vi "alpha_0.4.vi"() -> ()   [LabVIEW 2019]
panel:
  out "Congestionamento 2":bool
  in  "Rácio de entrada 2":dbl
  in  "Slide 2":dbl(slide) scale=0.0..10.0
  in  "Velocidade 2":dbl
  out "Vel3":bool
  out "Vel2":bool
  out "Vel1":bool
  out "RP1 3":bool
  out "GP1 3":bool
  out "G1 3":bool
  out "Y1 3":bool
  out "R1 3":bool
  out "RP1 2":bool
  out "GP1 2":bool
  out "G1 2":bool
  out "Y1 2":bool
  out "R1 2":bool
  out "RP1":bool
  out "GP1":bool
  out "G1":bool
  out "Y1":bool
  out "R1":bool
  in  "Rácio de entrada":dbl
  in  "Rácio de entrada 3":dbl
  out "Tempo no Vermelho":dbl caption="Elapsed Time (s)"
  out "Tempo no Verde + Amarelo":dbl caption="Elapsed Time (s)"
  out "Congestionamento 3":bool
  out "Congestionamento 1":bool
  in  "Slide 3":dbl(slide) scale=0.0..10.0
  in  "Slide 1":dbl(slide) scale=0.0..10.0
  in  "Caso de emergência":bool
  out "GreenP 2":bool
  out "RedP 2":bool
  out "GreenP 1":bool
  out "RedP 1":bool
  in  "Estado 2":dbl
  out "Velocidade excedida 3":bool
  in  "Velocidade 3":dbl
  out "RED 4":bool
  out "YELLOW 4":bool
  out "GREEN 4":bool
  out "Velocidade excedida 2":bool
  in  "Velocidade":dbl
  out "RED 3":bool
  out "YELLOW 3":bool
  out "GREEN 3":bool
  in  "stop":bool
  in  "Timer (s)":dbl
  # "Inputs"
  # "Inputs"
  # "Inputs"
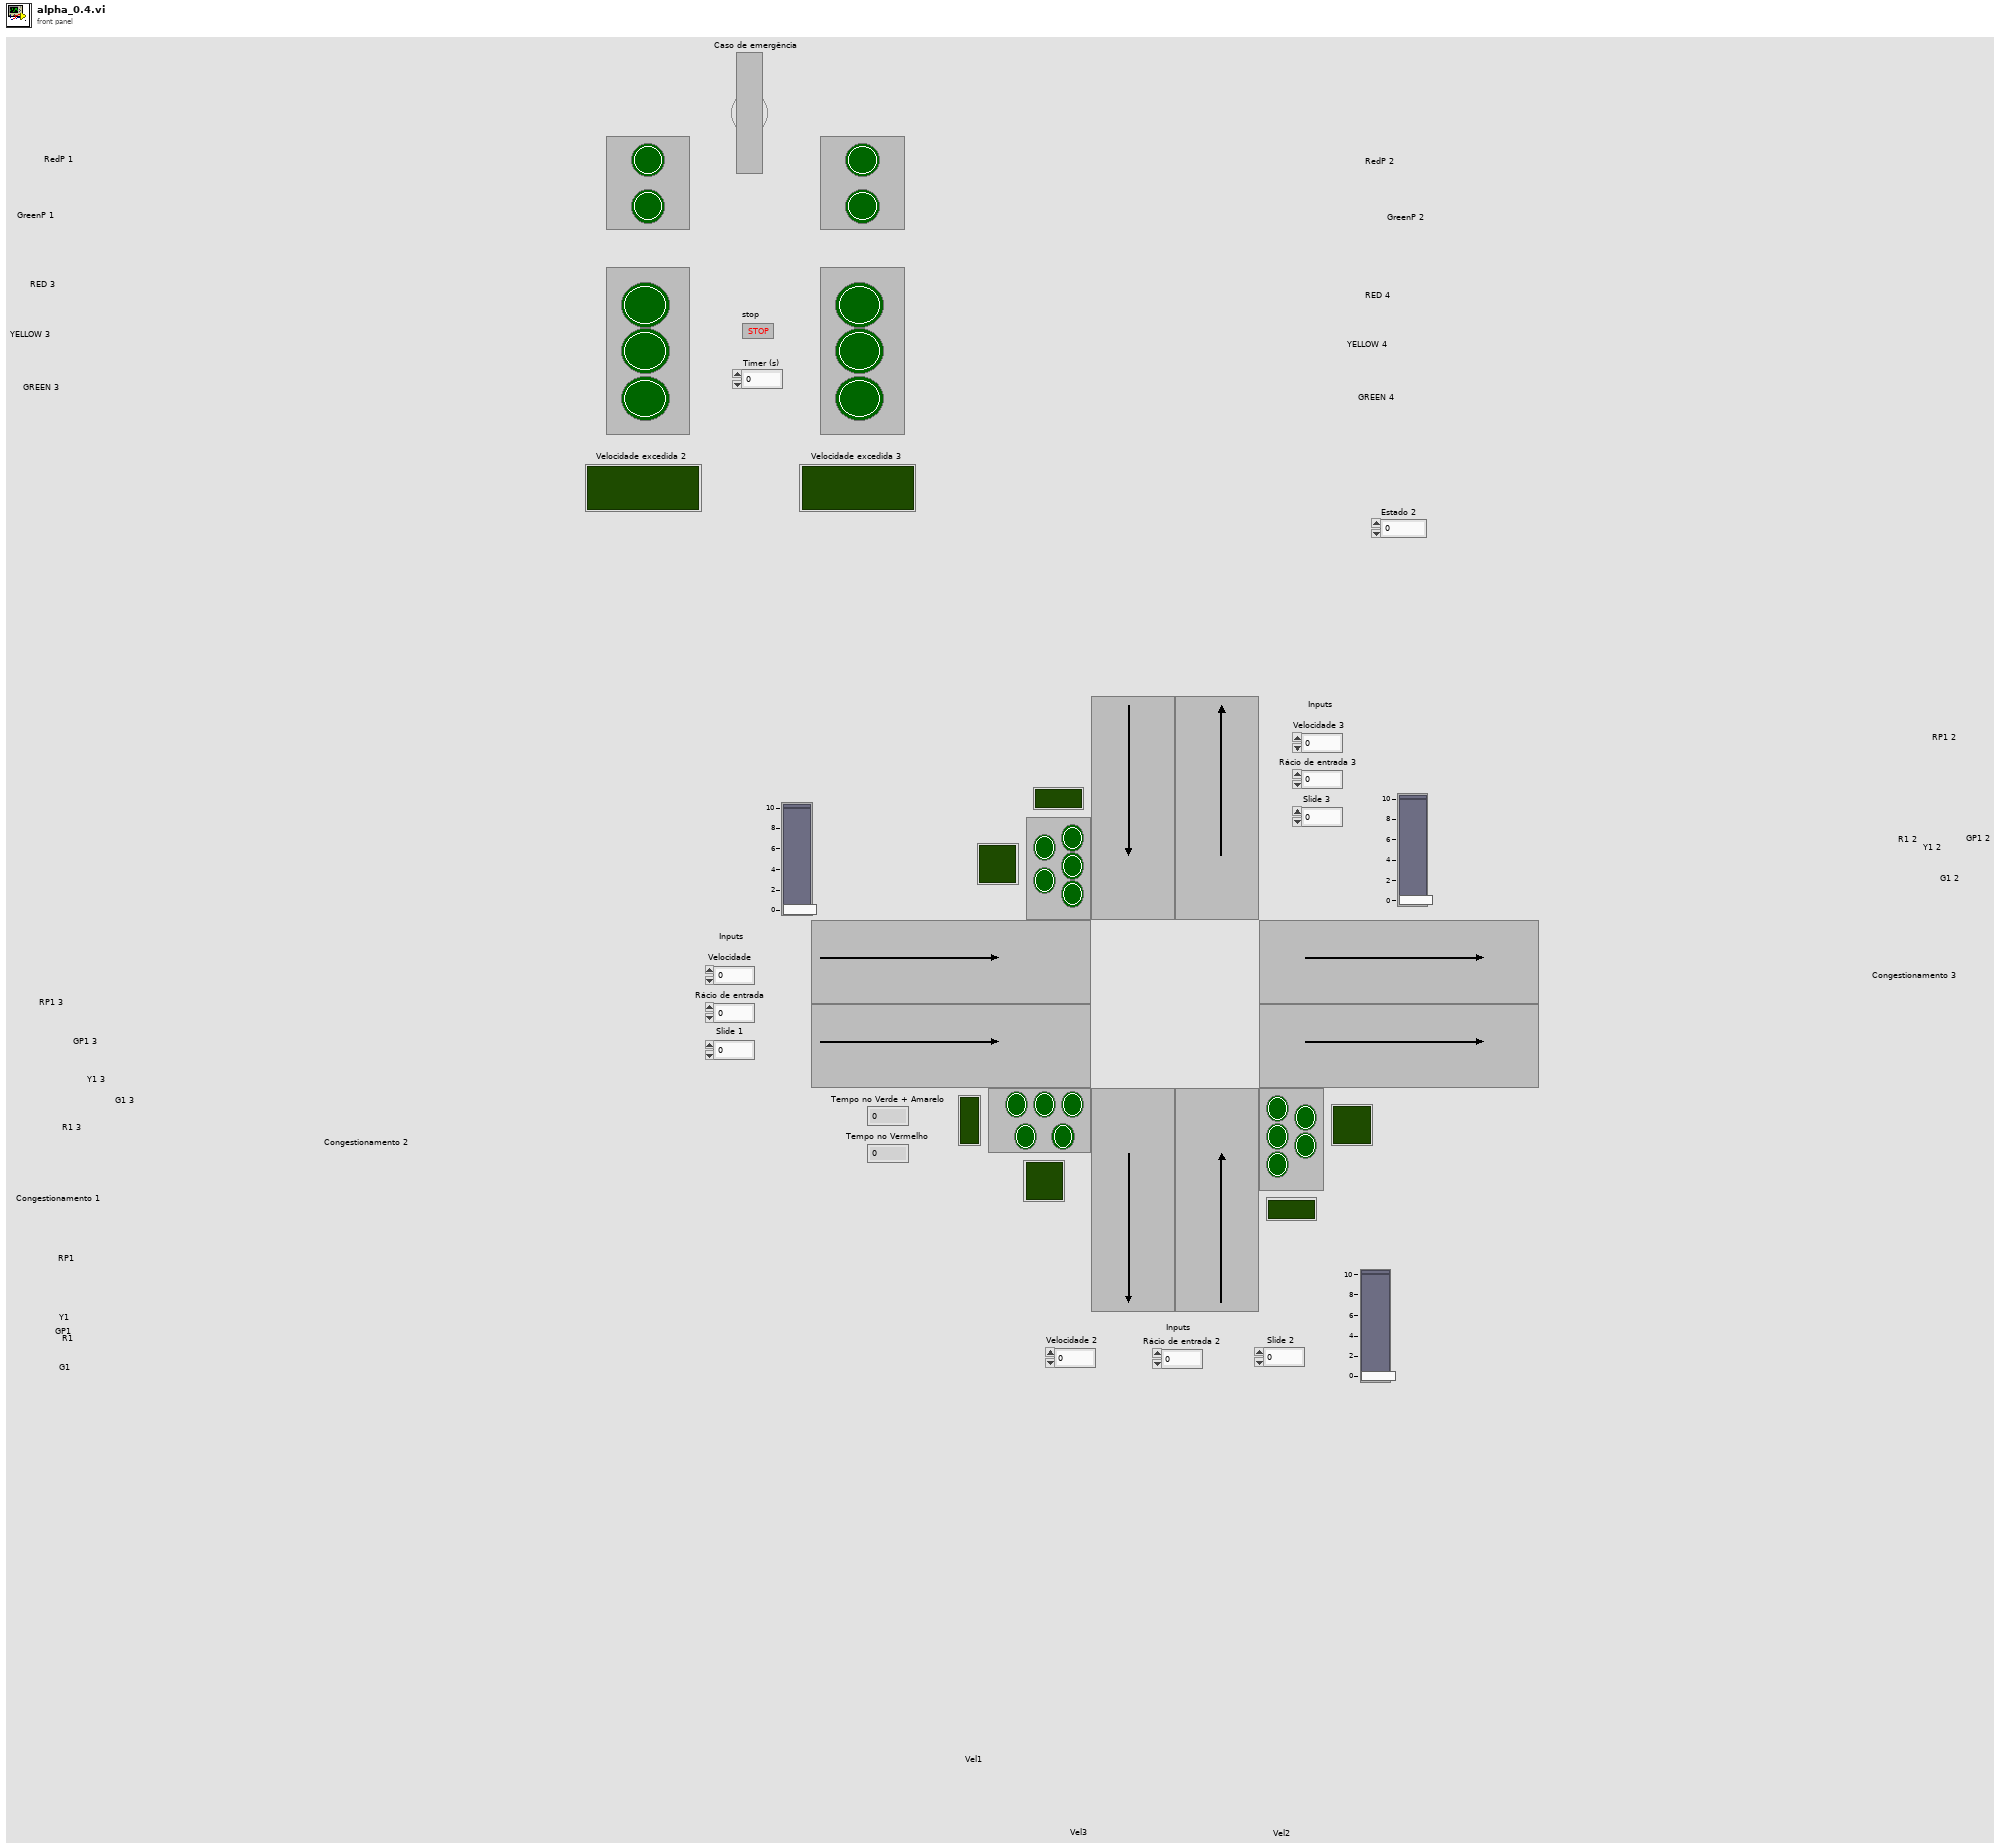
[diagram p1: front panel]
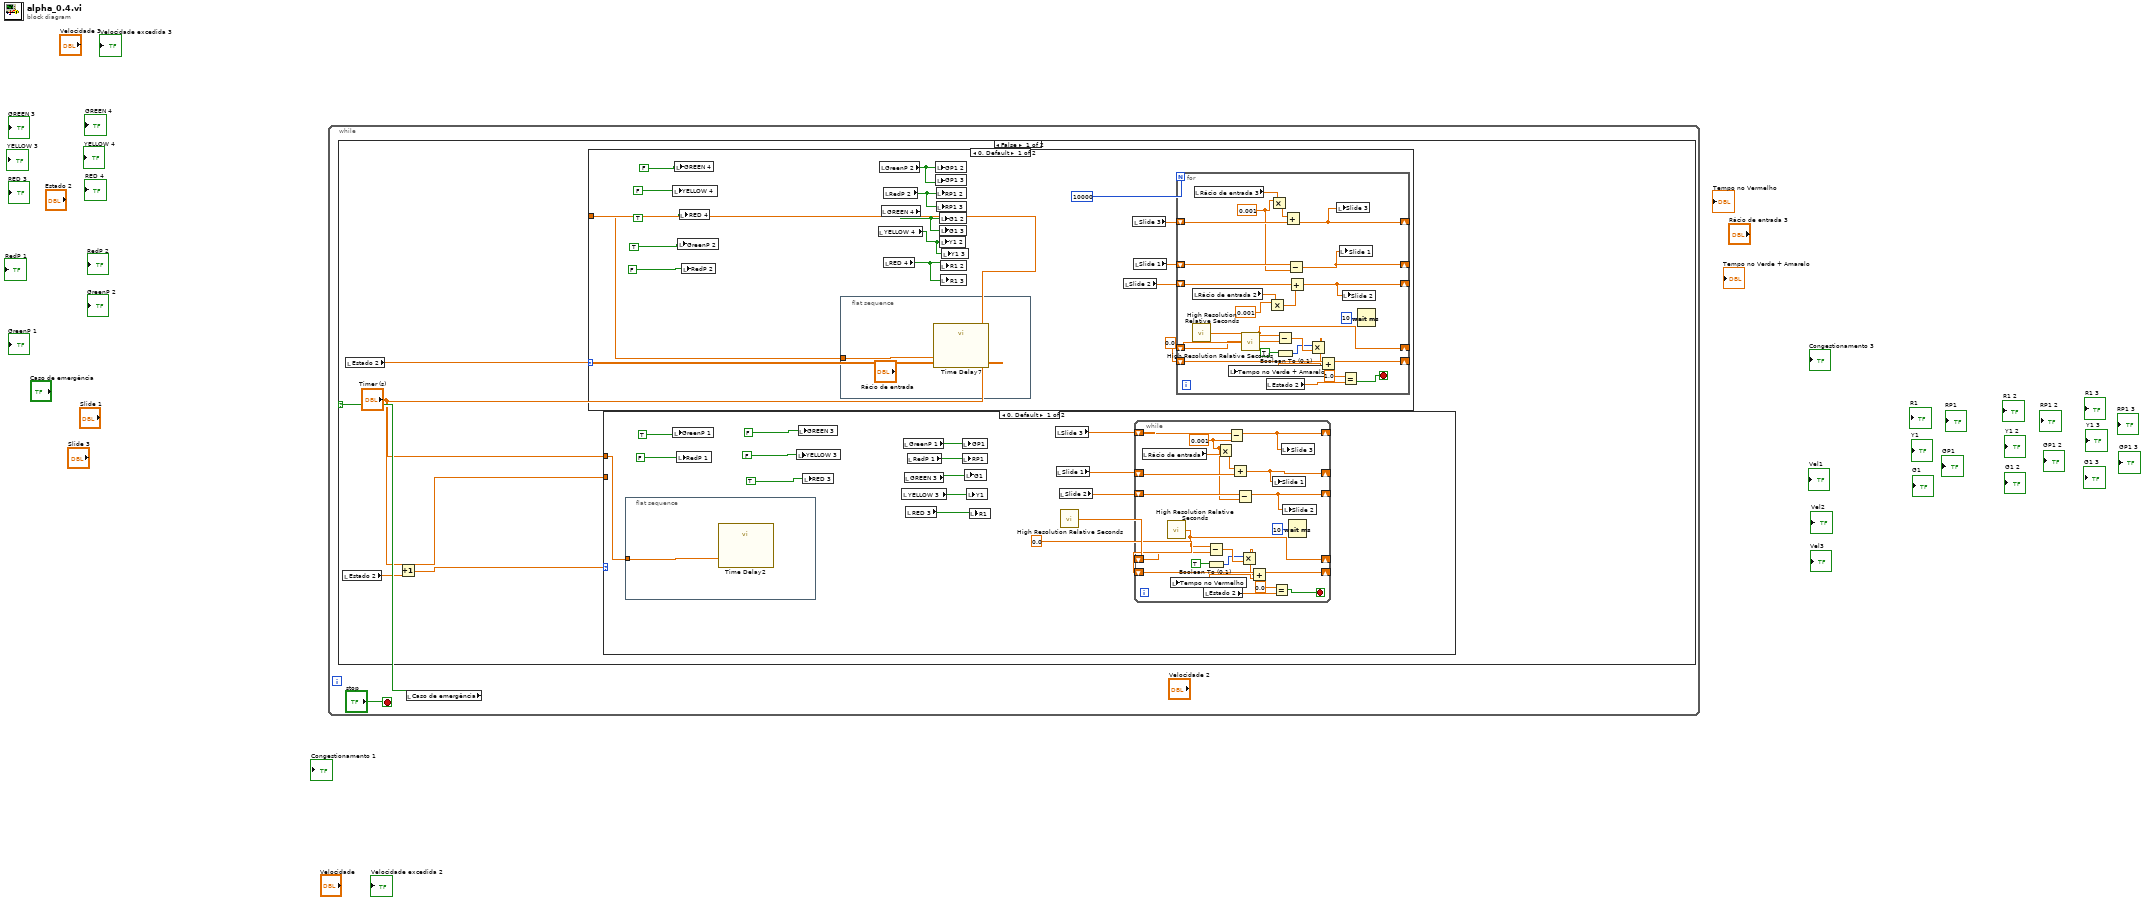
[diagram p0: block diagram]
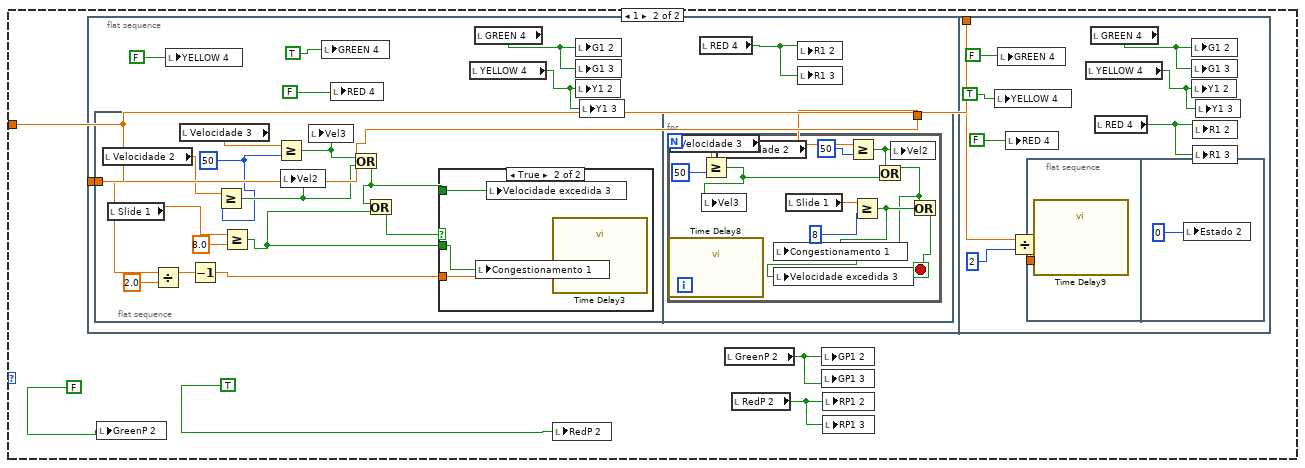
[diagram p2: hidden frame]
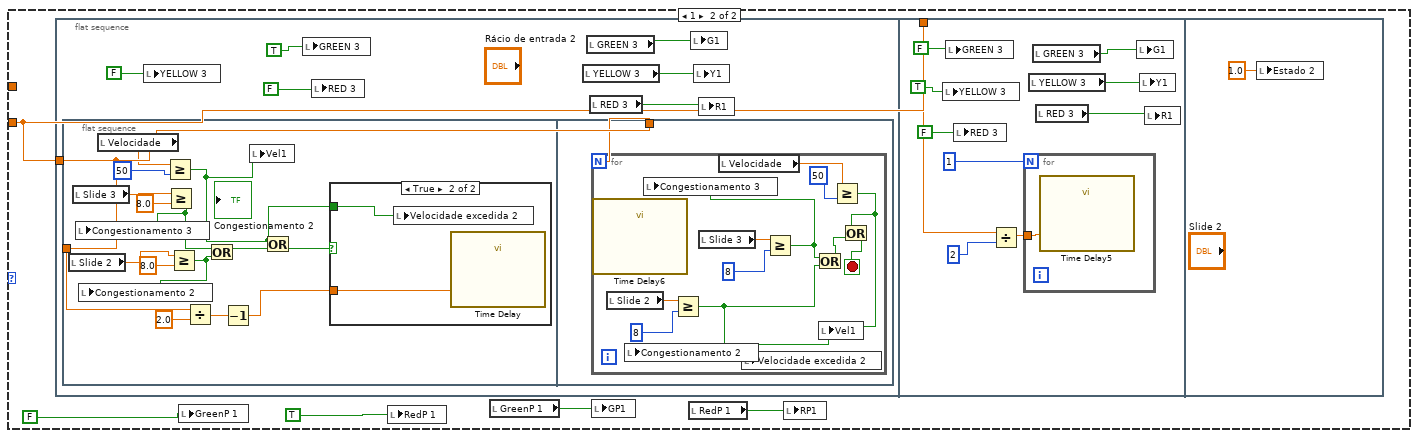
[diagram p4: hidden frame]
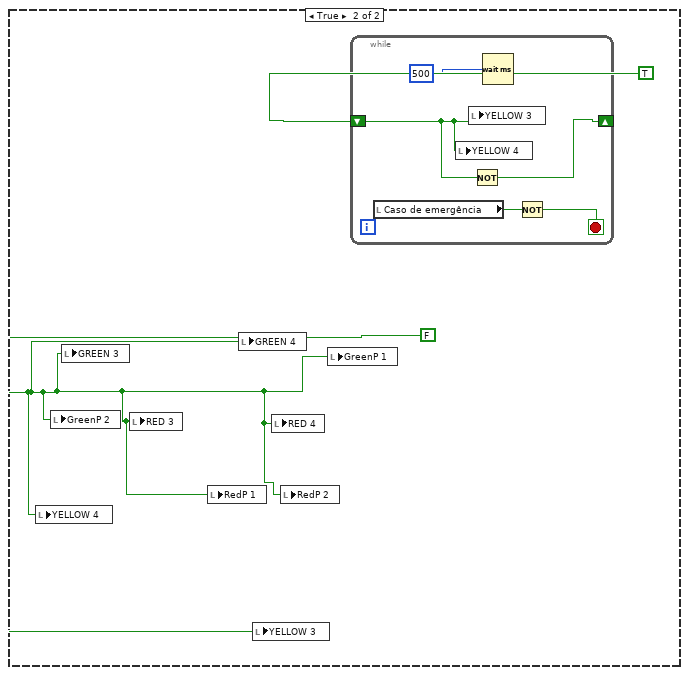
[diagram p6: hidden frame]
diagram:
  n1 = while {
    stop <- "stop" stop-if-true
    n2 = local read "Caso de emergência"() -> (w1:bool)
    n3 = case shown="False" w1 {
      frame False {
        n4 = local read "Estado 2"() -> (w6:dbl)
        n5 = local read "Estado 2"() -> (w4:dbl)
        n6 = Increment(x=w6) -> (x+1=w5:dbl)
        n7 = case shown="0, Default" w4 {
          tunnel: "Timer (s)" -> [w18 w53]
          frame 0, Default {
            n8 = local write "YELLOW 4"(FALSE) -> ()
            n9 = local write "GREEN 4"(FALSE) -> ()
            n10 = local write "GreenP 2"(TRUE) -> ()
            n11 = local write "RED 4"(TRUE) -> ()
            n12 = local write "RedP 2"(FALSE) -> ()
            n13 = flat-sequence {
              tunnel: w18 -> [w48]
              frame #0 {
                n14 = call "Time Delay7"("Delay Time (s)"=w48) -> ()  [unwired: 10 in, 1 out]
              }
            }
            n15 = local read "YELLOW 4"() -> (w9:bool)
            n16 = local read "GreenP 2"() -> (w12:bool)
            n17 = local read "GREEN 4"() -> (w10:bool)
            n18 = local read "RedP 2"() -> (w11:bool)
            n19 = local read "RED 4"() -> (w8:bool)
            n20 = local write "GP1 2"(w12) -> ()
            n21 = local write "GP1 3"(w12) -> ()
            n22 = local write "RP1 2"(w11) -> ()
            n23 = local write "RP1 3"(w11) -> ()
            n24 = local write "G1 2"(w10) -> ()
            n25 = local write "G1 3"(w10) -> ()
            n26 = local write "Y1 2"(w9) -> ()
            n27 = local write "R1 2"(w8) -> ()
            n28 = local write "R1 3"(w8) -> ()
            n29 = local write "Y1 3"(w9) -> ()
            n30 = local read "Slide 2"() -> (w7:dbl)
            n31 = local read "Slide 3"() -> (w13:dbl)
            n32 = local read "Slide 1"() -> (w14:dbl)
            n33 = call <vilib>:"High Resolution Relative Seconds.vi"() -> ("relative seconds"=w17:dbl)
            n34 = for {
              N: 10000 -> [_]
              shift-right: [w45] -> _
              shift-left: w17 -> [w46]
              shift-right: [w39] -> _
              shift-left: 0.0 -> [w44]
              shift-right: [w33] -> _
              shift-left: w13 -> [w35]
              shift-right: [w31] -> _
              shift-left: w14 -> [w30]
              shift-right: [w24] -> _
              shift-left: w7 -> [w28]
              stop <- w37 stop-if-true
              w29 = 0.001 ("x")
              n35 = local read "Rácio de entrada 2"() -> (w26:dbl)
              n36 = call <vilib>:"High Resolution Relative Seconds.vi"() -> ("relative seconds"=w45:dbl)
              n37 = local read "Rácio de entrada 3"() -> (w34:dbl)
              n38 = local read "Estado 2"() -> (w38:dbl)
              n39 = Multiply(x=0.001, y=w26) -> (x*y=w25:dbl)
              n40 = Multiply(x=w29, y=w34) -> (x*y=w32:dbl)
              n41 = Subtract(x=w45, y=w46) -> (x-y=w42:dbl)
              n42 = Boolean To (0,1)(Boolean=TRUE) -> (0, 1=w40:i16)
              n43 = Add(x=w32, y=w35) -> (x+y=w33:dbl)
              n44 = Subtract(x=w30, y=w29) -> (x-y=w31:dbl)
              n45 = Add(x=w28, y=w25) -> (x+y=w24:dbl)
              n46 = Multiply(x=w40, y=w42) -> (x*y=w41:dbl)
              n47 = Add(x=w44, y=w41) -> (x+y=w39:dbl)
              n48 = local write "Tempo no Verde + Amarelo"(w39) -> ()
              n49 = local write "Slide 3"(w33) -> ()
              n50 = local write "Slide 1"(w31) -> ()
              n51 = Equal?(x=1.0, y=w38) -> (x = y?=w37:bool)
              n52 = local write "Slide 2"(w24) -> ()
              n53 = Wait (ms)(milliseconds to wait=u32 10) -> ()  [unwired: 1 out]
            }
          }
          frame 1 {
            n54 = flat-sequence {
              tunnel: w53 -> [w57]
              tunnel: w53 -> [w94]
              frame #0 {
                n55 = flat-sequence {
                  tunnel: w57 -> [w70]
                  tunnel: w57 -> [w78]
                  frame #0 {
                    w61 = 50
                    n56 = local read "Velocidade 2"() -> (w63:dbl)
                    n57 = local read "Slide 1"() -> (w67:dbl)
                    n58 = Divide(x=w70, y=2.0) -> (x/y=w73:dbl)
                    n59 = local read "Velocidade 3"() -> (w72:dbl)
                    n60 = Decrement(x=w73) -> (x-1=w74:dbl)
                    n61 = Greater Or Equal?(x=w63, y=w61) -> (x >= y?=w62:bool)
                    n62 = Greater Or Equal?(x=w67, y=8.0) -> (x >= y?=w65:bool)
                    n63 = Greater Or Equal?(x=w72, y=w61) -> (x >= y?=w66:bool)
                    n64 = local write "Vel2"(w62) -> ()
                    n65 = local write "Vel3"(w66) -> ()
                    n66 = Or(x=w66, y=w62) -> (x .or. y?=w64:bool)
                    n67 = Or(x=w64, y=w65) -> (x .or. y?=w68:bool)
                    n68 = case shown="True" w68 {
                      tunnel: w74 -> [_ w77]
                      tunnel: w64 -> [_ w75]
                      tunnel: w65 -> [_ w76]
                      frame False {
                      }
                      frame True {
                        n69 = local write "Congestionamento 1"(w76) -> ()
                        n70 = local write "Velocidade excedida 3"(w75) -> ()
                        n71 = call "Time Delay3"("Delay Time (s)"=w77) -> ()  [unwired: 10 in, 1 out]
                      }
                    }
                  }
                  frame #1 {
                    n72 = for {
                      N: w78 -> [_]
                      stop <- w87 stop-if-true
                      n73 = call "Time Delay8"() -> ()  [unwired: 11 in, 1 out]
                      n74 = local read "Velocidade 3"() -> (w89:dbl)
                      n75 = Greater Or Equal?(x=w89, y=50) -> (x >= y?=w83:bool)
                      n76 = local write "Vel3"(w83) -> ()
                      n77 = local read "Velocidade 2"() -> (w81:dbl)
                      n78 = local read "Slide 1"() -> (w86:dbl)
                      n79 = Greater Or Equal?(x=w81, y=50) -> (x >= y?=w79:bool)
                      n80 = Greater Or Equal?(x=w86, y=8) -> (x >= y?=w84:bool)
                      n81 = local write "Congestionamento 1"(w84) -> ()
                      n82 = Or(x=w79, y=w83) -> (x .or. y?=w82:bool)
                      n83 = local write "Velocidade excedida 3"(w82) -> ()
                      n84 = local write "Vel2"(w79) -> ()
                      n85 = Or(x=w82, y=w84) -> (x .or. y?=w87:bool)
                    }
                  }
                }
                n86 = local write "YELLOW 4"(FALSE) -> ()
                n87 = local write "GREEN 4"(TRUE) -> ()
                n88 = local write "RED 4"(FALSE) -> ()
                n89 = local read "YELLOW 4"() -> (w55:bool)
                n90 = local read "GREEN 4"() -> (w56:bool)
                n91 = local write "G1 2"(w56) -> ()
                n92 = local write "G1 3"(w56) -> ()
                n93 = local write "Y1 2"(w55) -> ()
                n94 = local write "Y1 3"(w55) -> ()
                n95 = local read "RED 4"() -> (w54:bool)
                n96 = local write "R1 2"(w54) -> ()
                n97 = local write "R1 3"(w54) -> ()
              }
              frame #1 {
                n98 = local write "YELLOW 4"(TRUE) -> ()
                n99 = local write "GREEN 4"(FALSE) -> ()
                n100 = local write "RED 4"(FALSE) -> ()
                n101 = Divide(x=w94, y=2) -> (x/y=w93:dbl)
                n102 = flat-sequence {
                  tunnel: w93 -> [w99]
                  frame #0 {
                    n103 = call "Time Delay9"("Delay Time (s)"=w99) -> ()  [unwired: 10 in, 1 out]
                  }
                  frame #1 {
                    n104 = local write "Estado 2"(0) -> ()
                  }
                }
                n105 = local read "YELLOW 4"() -> (w91:bool)
                n106 = local read "GREEN 4"() -> (w92:bool)
                n107 = local read "RED 4"() -> (w90:bool)
                n108 = local write "G1 2"(w92) -> ()
                n109 = local write "G1 3"(w92) -> ()
                n110 = local write "Y1 2"(w91) -> ()
                n111 = local write "R1 2"(w90) -> ()
                n112 = local write "R1 3"(w90) -> ()
                n113 = local write "Y1 3"(w91) -> ()
              }
            }
            n114 = local write "GreenP 2"(FALSE) -> ()
            n115 = local write "RedP 2"(TRUE) -> ()
            n116 = local read "GreenP 2"() -> (w50:bool)
            n117 = local read "RedP 2"() -> (w49:bool)
            n118 = local write "GP1 2"(w50) -> ()
            n119 = local write "GP1 3"(w50) -> ()
            n120 = local write "RP1 2"(w49) -> ()
            n121 = local write "RP1 3"(w49) -> ()
          }
        }
        n122 = case shown="0, Default" w5 {
          tunnel: "Timer (s)" -> [_ w141]
          tunnel: "Timer (s)" -> [w108 _]
          frame 0, Default {
            n123 = flat-sequence {
              tunnel: w108 -> [w117]
              frame #0 {
                n124 = call "Time Delay2"("Delay Time (s)"=w117) -> ()  [unwired: 10 in, 1 out]
              }
            }
            n125 = local write "GreenP 1"(TRUE) -> ()
            n126 = local write "RedP 1"(FALSE) -> ()
            n127 = local write "YELLOW 3"(FALSE) -> ()
            n128 = local write "GREEN 3"(FALSE) -> ()
            n129 = local write "RED 3"(TRUE) -> ()
            n130 = local read "YELLOW 3"() -> (w103:bool)
            n131 = local read "GreenP 1"() -> (w106:bool)
            n132 = local read "GREEN 3"() -> (w104:bool)
            n133 = local read "RED 3"() -> (w102:bool)
            n134 = local read "RedP 1"() -> (w105:bool)
            n135 = local write "GP1"(w106) -> ()
            n136 = local write "RP1"(w105) -> ()
            n137 = local write "G1"(w104) -> ()
            n138 = local write "Y1"(w103) -> ()
            n139 = local write "R1"(w102) -> ()
            n140 = local read "Slide 3"() -> (w109:dbl)
            n141 = local read "Slide 1"() -> (w107:dbl)
            n142 = local read "Slide 2"() -> (w101:dbl)
            n143 = call <vilib>:"High Resolution Relative Seconds.vi"() -> ("relative seconds"=w111:dbl)
            n144 = while {
              shift-right: [w136] -> _
              shift-left: w111 -> [w137]
              shift-right: [w130] -> _
              shift-left: 0.0 -> [w135]
              shift-right: [w125] -> _
              shift-left: w109 -> [w126]
              shift-right: [w121] -> _
              shift-left: w107 -> [w122]
              shift-right: [w119] -> _
              shift-left: w101 -> [w120]
              stop <- w128 stop-if-true
              w118 = 0.001 ("y")
              n145 = local read "Rácio de entrada"() -> (w124:dbl)
              n146 = call <vilib>:"High Resolution Relative Seconds.vi"() -> ("relative seconds"=w136:dbl)
              n147 = local read "Estado 2"() -> (w129:dbl)
              n148 = Subtract(x=w136, y=w137) -> (x-y=w133:dbl)
              n149 = Boolean To (0,1)(Boolean=TRUE) -> (0, 1=w131:i16)
              n150 = Multiply(x=w118, y=w124) -> (x*y=w123:dbl)
              n151 = Subtract(x=w126, y=w118) -> (x-y=w125:dbl)
              n152 = Add(x=w123, y=w122) -> (x+y=w121:dbl)
              n153 = Subtract(x=w120, y=w118) -> (x-y=w119:dbl)
              n154 = Multiply(x=w131, y=w133) -> (x*y=w132:dbl)
              n155 = Add(x=w135, y=w132) -> (x+y=w130:dbl)
              n156 = local write "Tempo no Vermelho"(w130) -> ()
              n157 = local write "Slide 1"(w121) -> ()
              n158 = Equal?(x=0.0, y=w129) -> (x = y?=w128:bool)
              n159 = local write "Slide 3"(w125) -> ()
              n160 = local write "Slide 2"(w119) -> ()
              n161 = Wait (ms)(milliseconds to wait=u32 10) -> ()  [unwired: 1 out]
            }
          }
          frame 1 {
            n162 = flat-sequence {
              tunnel: w141 -> [w147]
              tunnel: w141 -> [w183]
              frame #0 {
                n163 = flat-sequence {
                  tunnel: w147 -> [w163]
                  tunnel: w147 -> [w168]
                  frame #0 {
                    n164 = local read "Slide 2"() -> (w151:dbl)
                    n165 = local read "Slide 3"() -> (w158:dbl)
                    n166 = local read "Velocidade"() -> (w165:dbl)
                    n167 = Greater Or Equal?(x=w165, y=50) -> (x >= y?=w156:bool)
                    n168 = Greater Or Equal?(x=w158, y=8.0) -> (x >= y?=w155:bool)
                    n169 = local write "Congestionamento 3"(w155) -> ()
                    n170 = Greater Or Equal?(x=w151, y=8.0) -> (x >= y?=w152:bool)
                    n171 = local write "Congestionamento 2"(w152) -> ()
                    n172 = Divide(x=w163, y=2.0) -> (x/y=w162:dbl)
                    n173 = Or(x=w155, y=w152) -> (x .or. y?=w154:bool)
                    n174 = Decrement(x=w162) -> (x-1=w160:dbl)
                    n175 = local write "Vel1"(w156) -> ()
                    n176 = Or(x=w156, y=w154) -> (x .or. y?=w159:bool)
                    n177 = case shown="True" w159 {
                      tunnel: w160 -> [_ w167]
                      tunnel: w156 -> [_ w166]
                      frame False {
                      }
                      frame True {
                        n178 = local write "Velocidade excedida 2"(w166) -> ()
                        n179 = call "Time Delay"("Delay Time (s)"=w167) -> ()  [unwired: 10 in, 1 out]
                      }
                    }
                  }
                  frame #1 {
                    n180 = for {
                      N: w168 -> [_]
                      stop <- w175 stop-if-true
                      n181 = call "Time Delay6"() -> ()  [unwired: 11 in, 1 out]
                      n182 = local read "Slide 2"() -> (w172:dbl)
                      n183 = Greater Or Equal?(x=w172, y=8) -> (x >= y?=w169:bool)
                      n184 = local write "Congestionamento 2"(w169) -> ()
                      n185 = local read "Slide 3"() -> (w177:dbl)
                      n186 = local read "Velocidade"() -> (w179:dbl)
                      n187 = Greater Or Equal?(x=w177, y=8) -> (x >= y?=w170:bool)
                      n188 = local write "Congestionamento 3"(w170) -> ()
                      n189 = Or(x=w170, y=w169) -> (x .or. y?=w171:bool)
                      n190 = Greater Or Equal?(x=w179, y=50) -> (x >= y?=w174:bool)
                      n191 = local write "Velocidade excedida 2"(w174) -> ()
                      n192 = local write "Vel1"(w174) -> ()
                      n193 = Or(x=w174, y=w171) -> (x .or. y?=w175:bool)
                    }
                  }
                }
                n194 = local write "YELLOW 3"(FALSE) -> ()
                n195 = local write "GREEN 3"(TRUE) -> ()
                n196 = local write "RED 3"(FALSE) -> ()
                n197 = local read "YELLOW 3"() -> (w145:bool)
                n198 = local read "GREEN 3"() -> (w146:bool)
                n199 = local read "RED 3"() -> (w144:bool)
                n200 = local write "G1"(w146) -> ()
                n201 = local write "Y1"(w145) -> ()
                n202 = local write "R1"(w144) -> ()
              }
              frame #1 {
                n203 = local write "YELLOW 3"(TRUE) -> ()
                n204 = local write "GREEN 3"(FALSE) -> ()
                n205 = local write "RED 3"(FALSE) -> ()
                n206 = Divide(x=w183, y=2) -> (x/y=w186:dbl)
                n207 = for {
                  N: 1 -> [_]
                  tunnel: w186 -> [w190]
                  n208 = call "Time Delay5"("Delay Time (s)"=w190) -> ()  [unwired: 10 in, 1 out]
                }
                n209 = local read "YELLOW 3"() -> (w182:bool)
                n210 = local read "GREEN 3"() -> (w180:bool)
                n211 = local read "RED 3"() -> (w181:bool)
                n212 = local write "G1"(w180) -> ()
                n213 = local write "Y1"(w182) -> ()
                n214 = local write "R1"(w181) -> ()
              }
              frame #2 {
                n215 = local write "Estado 2"(1.0 ("Estado 2")) -> ()
              }
            }
            n216 = local write "GreenP 1"(FALSE) -> ()
            n217 = local write "RedP 1"(TRUE) -> ()
            n218 = local read "GreenP 1"() -> (w139:bool)
            n219 = local write "GP1"(w139) -> ()
            n220 = local read "RedP 1"() -> (w140:bool)
            n221 = local write "RP1"(w140) -> ()
          }
        }
      }
      frame True {
        w192 = FALSE
        n222 = local write "YELLOW 4"(w192) -> ()
        n223 = local write "GreenP 2"(w192) -> ()
        n224 = local write "GREEN 3"(w192) -> ()
        n225 = local write "RED 3"(w192) -> ()
        n226 = local write "RedP 1"(w192) -> ()
        n227 = local write "GREEN 4"(w192) -> ()
        n228 = local write "YELLOW 3"(w192) -> ()
        n229 = local write "RED 4"(w192) -> ()
        n230 = local write "RedP 2"(w192) -> ()
        n231 = local write "GreenP 1"(w192) -> ()
        n232 = while {
          shift-right: [w198] -> _
          shift-left: TRUE -> [w194]
          stop <- w195 stop-if-true
          n233 = local read "Caso de emergência"() -> (w196:bool)
          n234 = local write "YELLOW 4"(w194) -> ()
          n235 = local write "YELLOW 3"(w194) -> ()
          n236 = Not(x=w194) -> (.not. x?=w198:bool)
          n237 = Wait (ms)(milliseconds to wait=500) -> ()  [unwired: 1 out]
          n238 = Not(x=w196) -> (.not. x?=w195:bool)
        }
      }
    }
  }
